vi "resume_.vi"(6 "nargs":i32, 8 "error in (no error)":errorcluster, 11 "Lua in":refnum<class "Lua.lvclass">) -> (0 "error out":errorcluster, 1 "done?":bool, 3 "Lua out":refnum<class "Lua.lvclass">, 4 "nresults":i32)   [LabVIEW 2020, in "Lua for LabVIEW.lvlib" / "Lua.lvclass"]
doc: "Starts and resumes a coroutine in the given thread L.\n\nTo start a coroutine, you push onto the thread stack the main function plus any arguments; then you call lua_resume, with nargs being the number of arguments. This call returns when the coroutine suspends or finishes its execution. When it returns, the stack contains all values passed to lua_yield, or all values returned by the body function. lua_resume returns LUA_YIELD if the coroutine yields, LUA_OK if the coroutine finishes its execution without errors, or an error code in case of errors (see lua_pcall).\n\nIn case of errors, the stack is not unwound, so you can use the debug API over it. The error object is on the top of the stack.\n\nTo resume a coroutine, you remove any results from the last lua_yield, put on its stack only the values to be passed as results from yield, and then call lua_resume.\n\nThe parameter from represents the coroutine that is resuming L. If there is no such coroutine, this parameter can be NULL."
uses:
  Lua.lvclass
  Lua.lvclass/Lua.ctl
  lib/lua.dll/lua_tolstring.vi
  lib/lua.dll/lua_pop.vi
  lib/lua.dll/lua_settop.vi
  lib/lua.dll/lua.dll.lvlib
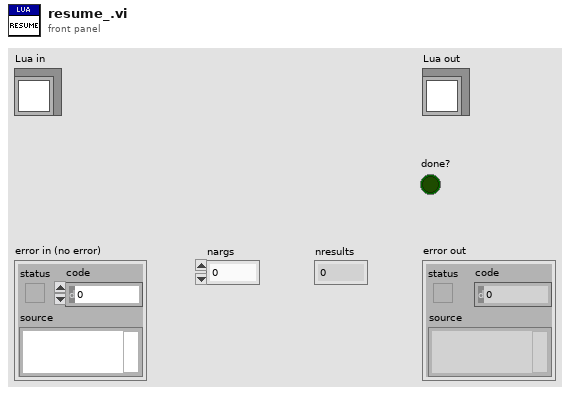
[diagram p1: front panel]
types:
  T1 = typedef "lua.dll.lvlib/lua_types.ctl" = i32
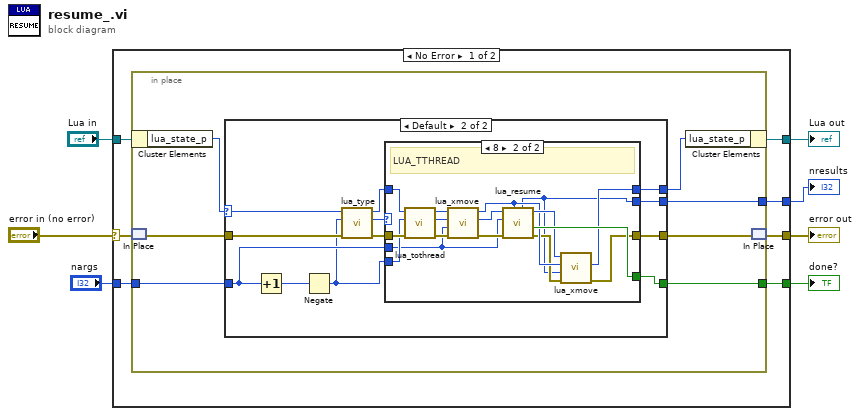
[diagram p0: block diagram]
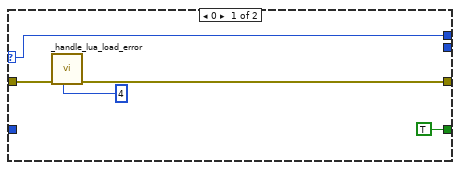
[diagram p2: hidden frame]
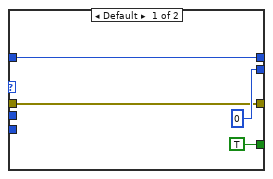
[diagram p3: hidden frame]
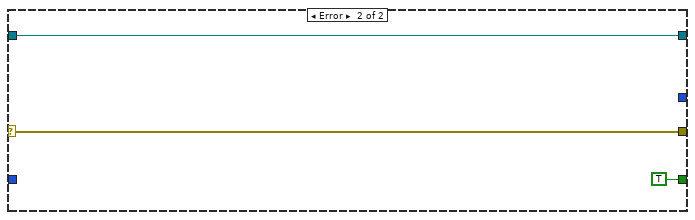
[diagram p4: hidden frame]
diagram:
  n1 = case shown="No Error" "error in (no error)" {
    selector: "error in (no error)" -> [w11 w61]
    tunnel: [w12 w61] -> w4
    tunnel: [w13 w60] -> w7
    tunnel: "Lua in" -> [w14 w60]
    tunnel: "nargs" -> [w10 _]
    tunnel: [w9 _] -> w2
    tunnel: [w8 TRUE ("done?")] -> w1
    frame No Error {
      n2 = in-place {
        in-place-border: w10 -> [w17]
        in-place-border: [w16] -> w9
        in-place-border: [w15] -> w8
        n3 = in-place-cluster #1(w14) -> ("lua_state_p"=w20:u64)
        n4 = in-place-match #2(w11) -> (w19:errorcluster)
        n5 = case shown="Default" w20 {
          selector: w20 -> [w26 w30]
          tunnel: [w26 w38] -> w21
          tunnel: w19 -> [w23 w33]
          tunnel: [w24 w36] -> w18
          tunnel: w17 -> [_ w34]
          tunnel: [_ w35] -> w16
          tunnel: [TRUE ("done?") w37] -> w15
          frame 0 {
            n6 = call "_handle_lua_load_error.vi"("lua_load errcode"=4, "error in (no error)"=w23) -> ("error out"=w24:errorcluster)  [unwired: 9 in]
          }
          frame Default {
            n7 = Increment(x=w34) -> (x+1=w32:i32)
            n8 = Negate(x=w32) -> (-x=w28:i32)
            n9 = call "lua_type.vi"("error in (no error)"=w33, "index"=w28, "lua_state_p"=w30) -> ("error out"=w27:errorcluster, "lua type"=w31:T1, "lua_state_p out"=w29:u64)  [unwired: 6 in]
            n10 = case shown="8" w31 {
              tunnel: [w39 w46] -> w38
              tunnel: [TRUE ("done?") w58] -> w37
              tunnel: [w40 w44] -> w36
              tunnel: [0 ("nresults") w43] -> w35
              tunnel: w29 -> [w39 w56]
              tunnel: w34 -> [_ w49]
              tunnel: w27 -> [w40 w57]
              tunnel: w28 -> [_ w55]
              frame Default {
              }
              frame 8 {
                # "LUA_TTHREAD"
                n11 = call "lua_tothread.vi"("error in (no error)"=w57, "index"=w55, "lua_state_p"=w56) -> ("error out"=w53:errorcluster, "thread out (lua_state_p)"=w51:u64, "lua_state_p out"=w54:u64)  [unwired: 6 in]
                n12 = call "lua_xmove.vi"("error in (no error)"=w53, "n"=w49, "to lua_state_p"=w51, "from lua_state_p"=w54) -> ("error out"=w52:errorcluster, "to lua_state_p out"=w50:u64, "from lua_state_p out"=w47:u64)  [unwired: 5 in]
                n13 = call "lua_resume.vi"("from_p"=w47, "error in (no error)"=w52, "nargs"=w49, "lua_state_p"=w50) -> ("error out"=w45:errorcluster, "done?"=w58:bool, "lua_state_p out"=w48:u64, "nresults"=w43:i32)  [unwired: 4 in]
                n14 = call "lua_xmove.vi"("error in (no error)"=w45, "n"=w43, "to lua_state_p"=w47, "from lua_state_p"=w48) -> ("error out"=w44:errorcluster, "to lua_state_p out"=w46:u64)  [unwired: 5 in, 1 out]
              }
            }
          }
        }
        n15 = in-place-cluster #1("lua_state_p"=w21) -> (w13:refnum<class "Lua.lvclass">)
        n16 = in-place-match #2(w18) -> (w12:errorcluster)
      }
    }
    frame Error {
    }
  }
  "error out" <- w4
  "Lua out" <- w7
  "nresults" <- w2
  "done?" <- w1
